vi "Send.vi"(6 "Hold":bool, 8 "error in":errorcluster, 11 "Data":string="Send") -> (0 "error out":errorcluster)   [LabVIEW 2015, in "TCP.lvlib"]
uses:
  TCP.lvlib
  support/Message Queue/Message Queue.lvlib
  support/Message Queue/Enqueue Message (Single).vi
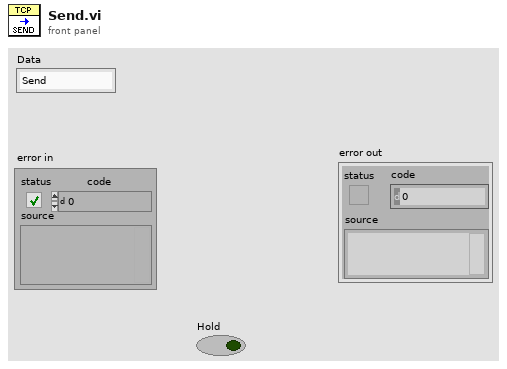
[diagram p1: front panel]
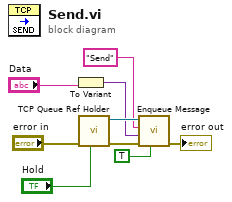
[diagram p0: block diagram]
diagram:
  n1 = To Variant(anything="Data") -> (Variant=w3:variant)
  n2 = call "TCP Queue Ref Holder.vi"("Hold"="Hold", "error in (no error)"="error in") -> ("error out"=w8:errorcluster, "Input Queue"=w5:refnum<queue>)  [unwired: 8 in]
  n3 = call-poly "Enqueue Message.vi"("Priority Message? (F)"=TRUE, "error in (no error)"=w8, "Message Data"=w3, "Message"="Send", "Message Queue"=w5) -> ("error out"=→"error out":errorcluster)  [unwired: 5 in, 1 out]
